vi "Update State.vi"(8 "Display State In":cluster{"Month":i32, "Day":i32, "Year":i32}, 10 "Data In":i32[](array[numeric])) -> (0 "Display State Out":cluster{"Month":i32, "Day":i32, "Year":i32})   [LabVIEW 2019, in "Custom Calendar.xctl"]
uses:
  Custom Calendar.xctl
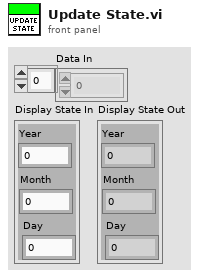
[diagram p1: front panel]
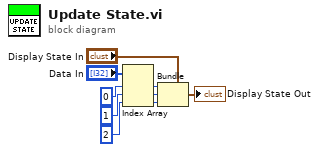
[diagram p0: block diagram]
diagram:
  n1 = Index Array(array="Data In", index #1=0 ("index"), index #2=1 ("index"), index #3=2 ("index")) -> (element #1=w4:i32, element #2=w3:i32, element #3=w2:i32)
  n2 = Bundle(cluster="Display State In", "Month"=w4, "Day"=w3, "Year"=w2) -> (→"Display State Out":cluster{"Month":i32, "Day":i32, "Year":i32})
